vi "VIve LabVIEW_menu_Properties.vi"(0 "Caption.button":string, 1 "reference":refnum<vi>, 7 "Button.name":string, 11 "Colors[4]":cluster{u32, u32}[](array[cluster])) -> (4 "Disabled":u8, 15 "error out":errorcluster)   [LabVIEW 2009]
doc: "Sets the preferences of a boolean button\n\nPreferences such as: Tip strip text, Disable, BoolText, Colors\n\nVIve LabVIEW"
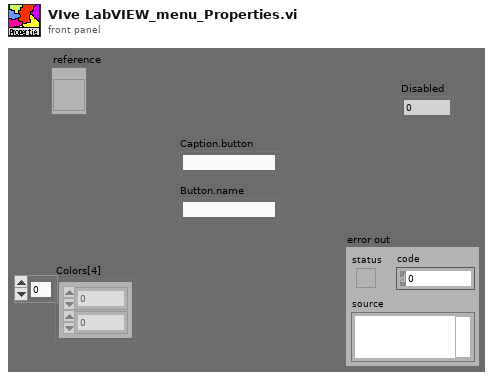
[diagram p1: front panel]
types:
  T1 = enum16{"Enable", "Disabled", "Disabled & Grayed"}
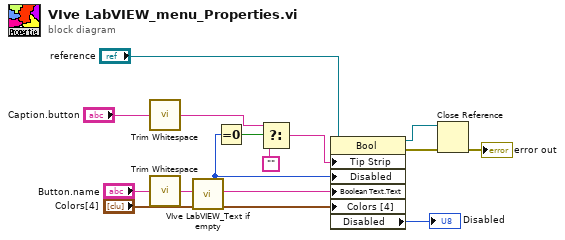
[diagram p0: block diagram]
diagram:
  n1 = call <vilib>:"Trim Whitespace.vi"("string"="Caption.button") -> ("trimmed string"=w6:string)  [unwired: 1 in]
  n2 = call <vilib>:"Trim Whitespace.vi"("string"="Button.name") -> ("trimmed string"=w14:string)  [unwired: 1 in]
  n3 = call "VIve LabVIEW_Text if empty.vi"("Text in"=w14) -> ("Property.Disabled"=w7:T1, "Text out"=w12:string)  [unwired: 17 in]
  n4 = Equal To 0?(x=w7) -> (x = 0?=w8:bool)
  n5 = Select(t=w6, s=w8, f="") -> (s? t:f=w5:string)
  n6 = property on="Property Node" class="Bool"(reference="reference", "Tip Strip"=w5, "Disabled"=w7, "Boolean Text.Text"=w12, "Colors [4]"="Colors[4]") -> (reference out=w3:refnum<vi>, error out=w2:errorcluster, "Disabled"=→"Disabled":u8)  [unwired: 1 in]
  n7 = Close Reference(reference=w3, error in (no error)=w2) -> (error out=→"error out":errorcluster)
